vi "3Decembre2016.vi"() -> ()   [LabVIEW 2014]
panel:
  out "Nb de triangle Partie 2":dbl
  out "Nb de Triangles 4":dbl
  out "Nb de Triangles 3":dbl
  out "Nb de Triangles 2":dbl
  out "Nb de Triangles":dbl
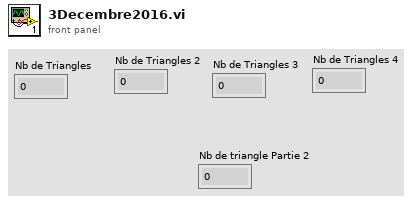
[diagram p1: front panel]
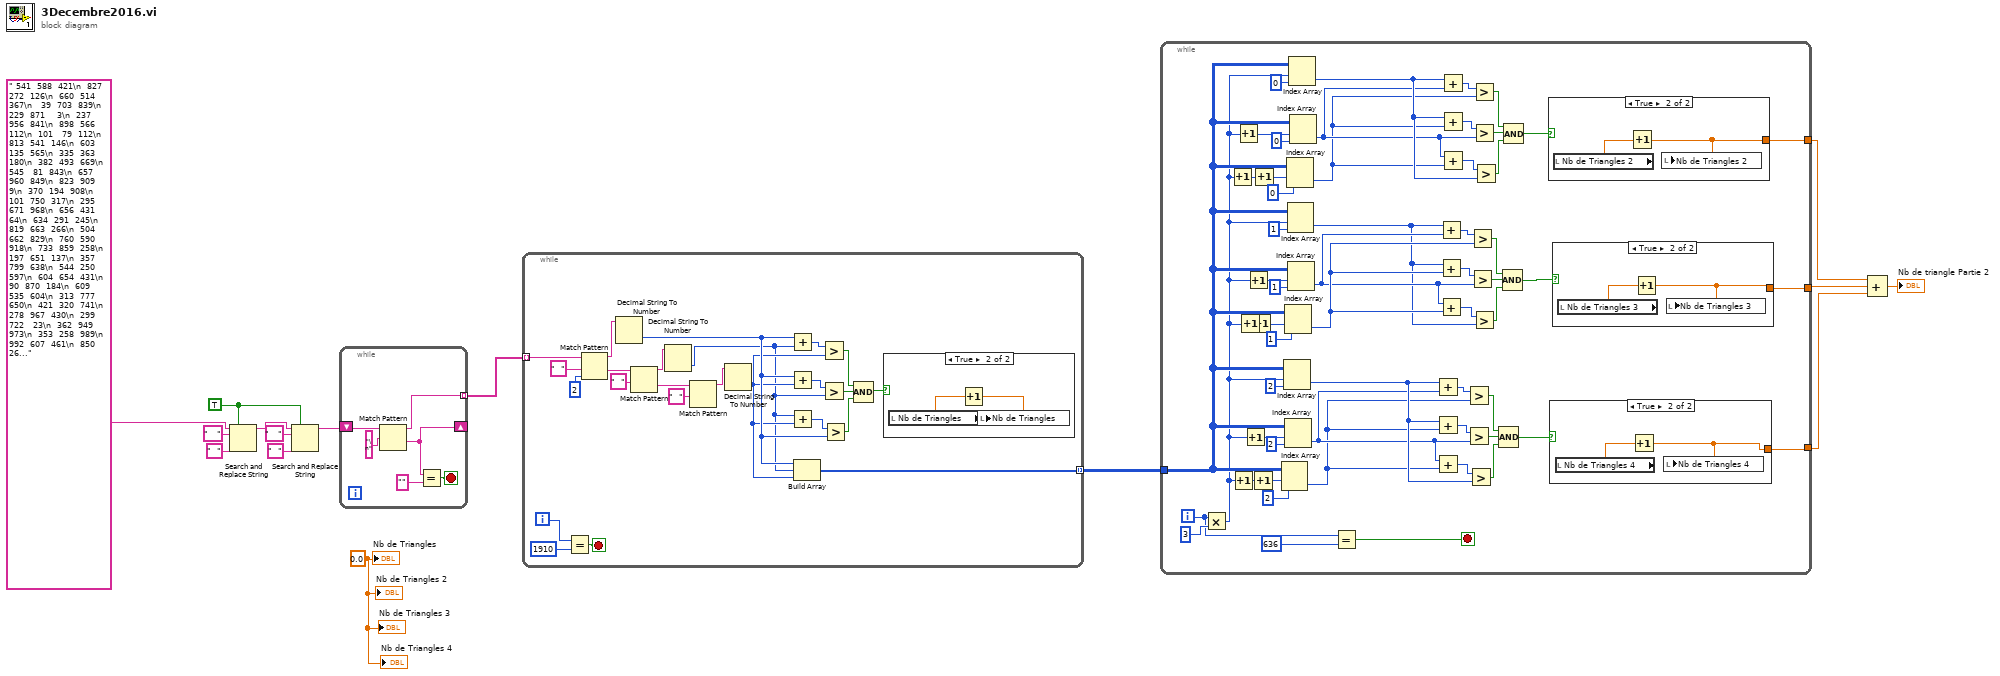
[diagram p0: block diagram]
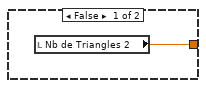
[diagram p2: hidden frame]
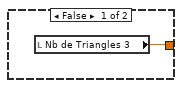
[diagram p3: hidden frame]
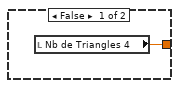
[diagram p4: hidden frame]
diagram:
  w1 = TRUE ("replace all? (F)")
  w14 = 0.0 ("Nb de Triangle")
  n1 = Search and Replace String(replace all?=w1, input string=" 541  588  421\n  827  272  126\n  660  514  367\n   39  703  839\n  229  871    3\n  237  956  841\n  898  566  112\n  101   79  112\n  813  541  146\n  603  135  565\n  335  363  180\n  382  493  669\n  545   81  843\n  657  960  849\n  823  909    9\n  370  194  908\n  101  750  317\n  295  671  968\n  656  431   64\n  634  291  245\n  819  663  266\n  504  662  829\n  760  590  918\n  733  859  258\n  197  651  137\n  357  799  638\n  544  250  597\n  604  654  431\n   90  870  184\n  609  535  604\n  313  777  650\n  421  320  741\n  278  967  430\n  299  722   23\n  362  949  973\n  353  258  989\n  992  607  461\n  850  264  490\n  251  351  569\n  810  320  116\n  959  335  611\n  450  242  624\n  849   26  376\n  419   42  222\n  995   14  291\n  711  174  615\n   17  982  961\n  722  895  941\n  920  161  480\n  905  246  531\n  794  190  144\n  317  318  633\n  145  233  150\n  445  534  519\n  935  592  863\n  784  260  844\n  255  704  570\n  521   57   61\n  490  149  110\n  163  144  142\n  771  289   60\n  914  233  541\n  271   93  542\n  411  640  812\n  370  968   65\n   61  960  781\n  333   79  421\n  269  190  428\n  477  225   96\n  610  641  265\n  650  135  461\n  145  759  380\n  758  451  682\n  524  125  861\n  760  555  251\n  360  219  567\n  456  285  726\n  510   98  927\n  886  336  228\n  356  916  323\n  685  974  165\n  253  532  207\n  868  990  548\n  811  803  525\n  205  624  894\n  707  512  328\n  835  288  657\n  496  776  413\n  484  185   10\n   33  832  403\n  896  678  789\n  745  595  773\n  287  201  669\n  150  189  513\n  884   42  131\n  934  214  407\n  239  819  149\n  145  582  334\n  375  307  467\n  680   59  850\n  873  441  973\n  243  393  256\n  509  237  265\n  302  550  334\n  728  524  291\n  130  986  333\n   60  926  390\n  133  653  692\n  428  755  491\n   24  476  659\n  446  290  823\n  906  703  410\n  950  183  391\n  199  735  250\n  734  908  254\n  635  373   34\n  489  567  275\n  587  746  463\n  512  508  367\n  104  971  568\n  647  857  191\n  605   20  775\n  118  853  634\n  432  559  322\n  887  433  134\n  660  332  336\n  669  711  952\n  762  713  610\n  108  972  860\n  732  743  562\n  877  277  758\n  225  590  380\n  708   35  424\n  989  425  439\n  279  413  818\n  107  422  634\n  775  833  667\n  755  755  279\n  694  293    6\n  156   75  649\n  820  303  651\n  448  934  587\n   25  830  788\n  473  192  932\n  734  126  535\n  940  215  513\n  935  126  656\n  428  905  789\n  760  742  772\n  510  523  633\n  994  808  110\n   93  740  100\n  943   80  198\n  329  888  532\n   50  763  337\n  320  673  741\n  722   52  639\n   18  130  566\n  733  130  921\n  280  586  642\n  450  222  350\n  178  427  325\n  317  685  261\n  744  261  105\n  621  809  326\n  740  532  605\n  855  690  526\n  441  301  185\n  783  309  196\n  525  272  334\n  502   58  432\n  980  150  121\n  891  9  800\n  286  143  705\n  985  846  850\n  362  696   70\n  807  194  900\n  912  193  448\n  405  148  461\n  677  261   30\n  121  406  308\n   34  206  451\n  109  473  312\n   46  726  695\n  793  847   25\n  834  160  708\n  372  849  375\n  744  799  423\n  631  478  715\n  346   82  545\n  541  184   95\n  492  228  588\n  542  635   43\n   75  347  439\n  612  321  431\n  719  526  847\n  158  270  338\n  813  482  560\n  817  253  402\n  899  630  887\n  198  456  730\n  235  286  344\n  125  646  398\n  204  375  401\n   80  289  308\n  295  664  862\n  284  382  565\n  816  130  651\n  947  596  383\n  131  611  723\n  617  471  549\n  663  282  697\n  475  219  901\n  535  829  434\n  542  502  544\n   23  649  110\n  733  691  820\n  684   21  821\n  740  689    1\n  224  249  280\n  485  776  350\n  682  971  182\n  465   12  610\n  294  296   13\n  606  297  594\n  337  104    3\n  154  257  343\n  352  171  349\n  322  466  973\n  189  173  854\n  484  338  714\n  194  194  551\n  188  741  162\n   14  696  663\n  219  868   33\n  224  4  446\n  218  865  411\n  392  536  574\n  616  692  482\n  746  592   94\n  230   72  663\n  291  487   99\n  326  482  669\n  131  265  155\n   61  422  609\n   80  552  641\n  509  334  851\n  475  211  911\n  193  274  737\n  128   15  973\n  381   31  255\n  413   21  812\n  778  461    3\n  514  307  697\n  329  353  695\n   48   90  212\n  856  354  294\n  863  265  360\n  496  918  264\n  377  889  164\n  603  164  418\n  159  701  199\n  283  503  186\n  127  658   54\n  938  226  855\n  189  533  465\n  924  365  906\n  322  422  291\n  943  713  238\n  714  508  138\n  612  328   49\n  962  877  685\n  849  963  732\n  154  278  428\n   49  624  476\n  111  518  753\n  284  330  216\n  716  689  290\n  667  369  127\n  719  728  175\n  543  493  139\n  759  408  286\n  915  970  827\n  482  289  787\n  713  860  621\n  836  286  729\n  921  447  223\n  665  655  706\n  692  579  316\n  772  679  289\n  972  394   84\n  221  675  877\n  272  336  864\n  439  684   69\n  780  721  503\n  225  587  125\n  802  945  408\n  280  237  682\n  406  281  745\n  176   60   71\n  450  720  335\n  656  293  383\n  324  694  454\n  547   57   51\n  415  965  657\n  311  936  687\n  989  878  585\n  156   72  165\n  938  823  574\n  626  968  146\n  823  896  588\n  294  236  597\n  177  294  177\n  287  351  480\n  133  252  649\n  706  319  175\n   34  418  960\n  722  583  906\n  711  379  674\n  529  574  882\n  546  868  781\n  577  875  687\n  881  844  503\n  926  247  190\n  621  535  356\n  294  105  257\n  601  640  579\n  573  142  519\n  978  900  427\n  693  823  350\n  275  362  683\n  137  291  741\n  258  130  517\n  838  686   12\n   59  800  869\n  790  188  881\n  997  324  278\n  582  338  887\n  900   23  712\n  288  619  402\n  480  168  596\n  292  505  505\n  993   30  982\n  636  335  892\n  813  363  175\n  230  248  620\n  450  668  896\n  460  736  874\n  331  800  837\n  844  805  734\n  620   54  708\n  726  820  592\n  126   20  394\n  728  820  219\n  229   27   32\n  164  569  939\n  290  559  949\n  325  360  794\n  342  356  529\n  203  627  691\n   60  932  544\n  767  865  563\n  770  316  525\n   99  756  674\n  165  783  180\n   72   27  846\n  973  419  905\n  104  364  294\n  896  271  613\n  294  222  416\n  414  609  858\n  481  429  478\n  308  544  615\n  624  139  560\n  574  626  840\n  998  338  328\n  403  739  211\n  625  472  120\n  808  190  64\n  5  202  558\n  800   42  607\n  874  801  675\n   27  275  735\n  898  927  280\n  366  794  526\n  233  529   13\n  314  744  525\n  842  530  617\n  704  461  406\n  281  946  841\n  389  113  678\n  545  652  410\n  851  754  339\n   14   56  706\n  623  131  738\n  636  127  931\n  857  404  199\n  682   25  387\n  574  406  435\n  508  528  307\n  574  531  575\n  223  433  827\n   80  811  486\n  710  642  904\n  749  903  795\n  920  205   60\n  904  286  108\n   96  428  120\n  631  364  307\n  599  169  180\n  743  491  302\n  133  939  980\n  559  879  883\n  642  605  918\n  935  868  810\n  539  860  357\n  584  643  972\n  831  562  800\n  211  561  108\n  953  928  802\n  730  611   73\n  483  373  139\n  245  374  210\n  493  582   77\n  671  422  887\n  568  458  930\n  727  462  467\n  663  603  657\n  113  490  966\n   95   26  415\n   74   84  463\n  117   78  276\n   81  814  741\n  407  852   36\n  348   39  748\n  144   43  826\n  915  174  218\n  775  148  820\n  388  305  131\n  458  135  195\n  142  199   96\n   79  223  625\n  338   47  879\n  295  217  575\n  790   72  723\n  713  736  711\n  366  769  330\n  302  642  718\n  603  526  956\n  450  181  663\n  176  638  433\n  902  801  408\n  750  545   97\n  398  366  271\n  490  186  474\n  801  290  324\n  964  652  190\n  937  593  344\n  112  888  373\n  940  377  623\n  668  693  367\n  623  889  870\n  231  714  220\n  694  535  837\n  701  178  674\n  620  887   23\n  603  133  576\n  224  983  601\n  3  103  234\n  867  232   33\n  869  235  233\n  448  909  262\n  247  941  265\n  464  909    4\n   30  224   22\n  154   99  764\n  146  187  786\n  789  347  512\n  474  166  775\n  583  253  359\n  517  531  274\n  154  414  735\n  397  436  997\n  864  822  104\n  712  303  243\n  310  652  217\n  915  772  521\n   25  780  616\n  927  266  233\n  899  327  372\n  796  897  343\n  741  794  508\n  533  554  586\n  470  656  176\n  159  863  749\n  680  644  839\n  784  768  143\n  152  451  939\n  125  366   67\n  779  902  437\n  657  749  452\n  325  759  722\n  576  562  249\n  776  467  790\n  776  580  296\n  705  264   84\n  522  526  220\n  879  278  392\n  712  426  442\n  288  589  363\n   74   23  960\n  203  873   22\n  170  857  952\n  155   46   56\n  840  855  211\n  740  816  188\n  644  272  737\n  623  362  311\n  309  416  848\n  895  807  900\n  196  790  127\n  871  912  916\n  569  966  180\n  461  223  854\n  805  754  886\n  828  353  453\n  263  697  656\n  595  541  418\n  235  302  908\n  883  446  723\n  996  745  204\n  457  813  925\n  674  271  977\n  463  769   97\n  668  535  957\n  609  720  417\n  889  987  722\n  649  852  317\n  450   69  383\n  499  915  226\n  430  185  435\n  475  840  992\n  775  992  695\n  334  725  933\n  642  273  908\n  682  693   55\n   14  532  444\n   63  192  736\n   51  362  930\n  306  301  474\n  448  330  373\n  691  115  425\n  431  321  623\n  265  881  504\n  591  726  138\n   58  930  870\n  540  954  120\n  496  157  772\n  116  376  817\n  943  249  828\n  945  384  518\n  777  573  897\n  769  254  676\n  290  691  734\n  845  818  135\n  860  802   75\n  956  267  157\n  964   92  268\n  631  126  262\n  571   59   14\n   45  226  368\n  144  878  306\n  166  940  581\n  803   30   24\n   40  408  268\n  782  423  267\n  511  251  426\n  680  962  467\n  919  817  103\n  558  609  789\n  619    7  544\n  122  611  384\n  503  449   80\n  373  982  264\n  355  559  207\n  911  801  105\n  382  889  894\n  762  707  989\n  754   83  383\n  890  198  327\n  189  185  492\n  844  820  374\n  602  375   81\n  399  871  374\n  576  446  620\n  696  249  930\n  203  510  741\n  485  264   79\n  485  310  443\n  163  340  469\n  187   15  873\n  309  506  141\n  319  508  753\n  202  457  500\n  560  614  177\n  377  909  534\n   84   32  898\n  261  761  825\n  207  763   85\n  649  544  761\n  874  639  578\n  760  555  435\n  738  108  970\n  711  458  986\n   31  529   83\n   98  374  182\n  344  620  186\n  421  340   29\n  490  860  153\n   97  793  609\n  412   70  510\n  855  542  805\n  753  320  429\n  130  245  621\n  173  309   23\n  741  513  716\n  588  632  728\n   53  928  543\n  429  868  480\n  455   90  465\n  673  302  632\n  238  255  483\n  455   49  181\n  325  935  570\n  631  118  140\n  579  987  515\n  385  485  576\n  466  497   16\n   85   57  595\n  967  801  619\n  792  543  386\n  842  480  332\n  861  688  780\n   88  209  741\n  784  542  396\n  696  800  232\n  434  969  747\n  709  342  679\n  698  892  147\n  526  474  726\n  491  707  679\n  241  197  440\n  799  371  452\n  832  425   98\n  249  288  669\n  657  909  768\n  657  930  957\n  751  211  846\n  2  642  844\n  748  718   11\n  694  764  366\n  332  231  268\n  580  593  459\n  921  656  751\n  171  757  815\n  828  555  167\n   38  409  765\n  244  455  834\n  251  121  421\n  659  271  526\n  401  470  326\n  354  241  846\n  145  732  473\n   53  261  972\n  192  594  511\n  480  337  383\n   68  182  937\n  472  478  653\n   84  346  471\n  707  458  137\n  710  483  366\n  954   52  537\n  871  116  778\n  670  104  912\n  989  639  346\n  139  444  640\n  876  497  599\n  313    8  980\n  211  896  163\n  127  894  850\n  504  230   28\n  385  710   79\n  602  553   90\n  981  628  560\n  653  532  914\n  452  275  432\n  251  486  366\n  521  257  539\n  385  255  892\n  552  405  361\n  220  223  576\n  608  368  309\n  287   92  647\n   33  346  483\n  271  397  213\n  834    8  851\n  450  129   51\n  477  139  847\n  652  619  430\n  525  117  446\n  505  656  250\n  387   34  263\n  288  651  381\n  450  665  145\n  704  612  710\n  875  974  543\n  887  419  378\n  328  768  521\n  249   30  936\n  318  762  906\n  807  242   71\n  794  413  374\n  100  200  330\n  317   65  889\n  268  175  870\n   69  215  691\n  487  484  583\n  368  497  505\n  402   64  263\n  290  420  846\n  552  525  839\n  300  497  485\n  371  144  551\n  590  391  504\n  790  519  261\n  533  533  519\n  997  537  453\n  869   26  534\n  179  787  612\n  470    6  559\n  407  781  138\n  239  498  490\n  390  291  976\n  604  227  556\n   78  937  610\n  513  171  447\n  528  874  853\n  308  925   92\n  113  114  109\n  286  820  150\n   68   64  664\n   29  952  167\n   86  988  736\n  530  285   93\n  533  829  394\n  654  917  322\n   79  802  748\n   79  226  476\n   63  681  810\n  699  249   37\n  970  116   99\n  332  355   71\n  821  366  189\n  653  531  751\n  577  791  917\n  841  104  877\n  717  993  919\n  342  969   58\n  469  458  501\n  190  446  208\n  511  151  600\n  635  875  369\n  443  580  620\n  235  761  902\n  170  707  130\n  404  586  241\n  270  920  319\n  280  340  126\n  226  357  857\n  432  401  816\n  122  962  518\n  903  139   38\n  886  928  553\n  884  636  522\n  139  696  787\n  936  455  611\n  935  238  617\n  879  265  631\n  162  490  358\n  447  520  570\n  283  118  375\n  432  411  768\n  468  110   89\n  642  116  624\n  299    8  687\n  426  802  789\n  428  846  419\n   21  750  486\n  306  251  164\n  824   54  144\n  625  273  242\n  625  507  776\n  618  429  200\n  7  81  763\n  167  288   97\n   60  239  173\n  223  370  259\n  719  160  934\n  895  833   51\n  961  693  984\n  240  940  566\n  240  869  930\n  171  457  848\n  105  693  480\n  807  288  493\n  839  883  538\n   18  659  905\n  883  665  543\n  904  746  659\n  225  119  529\n  523  104  507\n  447   57  109\n  642  234  709\n  319  554  656\n  849  437  597\n  648  645  614\n  482  447  953\n  891  321  883\n  432  423  391\n  295  684  242\n  214  303  540\n  562  256  130\n  784  369  960\n  414  510  954\n  395  508  442\n  790  536  212\n  764  463  384\n  515   37  205\n  857  840  421\n  778  876  558\n  594  698  882\n  274  425  847\n  463  766  592\n  825  456  751\n   42  530  818\n  800  812  238\n  795  832  365\n  879  814  318\n  102  763  445\n  916  349  731\n  165  838  485\n  757  973  270\n  520  501  512\n  682  157  411\n  326  563  238\n  881  173  303\n  776  160  358\n  810  284  156\n  169  981  827\n  132  886  635\n  109  223  359\n  785   28  287\n  2  855  288\n  782  854   23\n  824  452  743\n  425   79  768\n  839  380  810\n  859  212  356\n  545  250  389\n  341  270   90\n  271   31  500\n  958   38  718\n  890    7  642\n  437  869  750\n  267  488  241\n  481  517  781\n  898  751  423\n  363  244    7\n  938  960  415\n  714  297  426\n  821  370  697\n  454   77  498\n  290  171  296\n  257  509  698\n  504  455  525\n  619  771  981\n  502  179  779\n  554  746  322\n  554  203  273\n  576  557   27\n  560  474  284\n   76   85   88\n  366  418  956\n  426  487  928\n  468  783  402\n  547  167  678\n  206  627  728\n  467  191  185\n  621  856  989\n  618  794  862\n  183  667  714\n  582  707  993\n  558   38  366\n  324  111  131\n  939  660  600\n  863  576  550\n  761  410  470\n  414  273  362\n  411  148  179\n  532  795  514\n  299  214  719\n  296  871  522\n  557  895   97\n  489  873  782\n  398   81  760\n  493   75  328\n  832  502   96\n  482  505  247\n  378  667   38\n  463  434   78\n  190  789   78\n  798  510  131\n  855  502  824\n  698  775  920\n  685  930  693\n  920  723  923\n  911  303  901\n  668  574  538\n  8  832  573\n  670  629  626\n  248  686   96\n  434  131  743\n  456  716  679\n  294  807  107\n  533  284  167\n  765  615  130\n  958  870  257\n  910  169  662\n  304  829  425\n  600  235  796\n  411  788  121\n  243  840  791\n  576  707  927\n  613  307  633\n   58  888  639\n  634  707  253\n  589  371  730\n  193  956  813\n  733  551  197\n  155  973  175\n  763  477  200\n  102  984   83\n  207  427  487\n  135  868  546\n  375  596  389\n  329  405  299\n  496  691  230\n  266  975  261\n  295  834  423\n   80  140  572\n  844  660  625\n  772   44  369\n  171  642  782\n  352  889  273\n  788  228  588\n  737  852  753\n  599  322  664\n  545  296  545\n  445  137  454\n  218   69  171\n  234  928  681\n   67  991  829\n  166  131  174\n  442   11  769\n  324  133  795\n  736  757  408\n   49  177  439\n  719  923   31\n  497  953  502\n  664  684  447\n  173  497  278\n  954  888  913\n  764  118  107\n  601  850  972\n  466   61   19\n  969  499  418\n  686  460  404\n  327  329  165\n  596  726  139\n  811  596   75\n  185  331  327\n  216  409  168\n  160  196  483\n  264  533    1\n  227  495  151\n  226  708  155\n  580  345  615\n  586  900  862\n   16  699  871\n   38  594  382\n  760  684  141\n  770  455  511\n  286  821  117\n  582  919  393\n  433  979  346\n   75  939  949\n  102  899  631\n   98  305  567\n  349  636  399\n  627  981  520\n  948  639  181\n  753  150  521\n  776  563  328\n   89  613  658\n  552  747  504\n  131  449  276\n  429  824  391\n  283  542  472\n  731  199  435\n  456  707  160\n  675  243  107\n  547  911  854\n  170  849  912\n  497  869  377\n  475  951  392\n  458  273   24\n  140  109  311\n   38  276  388\n  151  274  515\n  100  704  858\n  811  362   42\n  745  777  817\n  740  497   81\n  424  270  266\n  375  714  277\n  602  668  923\n   33  492  225\n  603  953  772\n  244   65  920\n  247  659   29\n  380  651  916\n  674  529  388\n  656  624  288\n   53  112  270\n  653  385  841\n  736  945  725\n  474  883  204\n  995   21  127\n  264  886  337\n  873  870  237\n  275   42  834\n  188  202  872\n  232  234  490\n  688  384   29\n  713  174  281\n   90  533  299\n  365  437  364\n  345  940  484\n  572  829  274\n  556  319   28\n  310  736   27\n  758  729   19\n  919  993  823\n  942  949  411\n  520  610  663\n  376   24  997\n  876  668  790\n  762  682  677\n  530  224  905\n  480  624  428\n  127  796  916\n  777  114  158\n   38  824  844\n  771  821  741\n  870  738  438\n  615   13  677\n  856  751  710\n   68   89  515\n  827  390  728\n  889  356  930\n  741  935  128\n  858  515  386\n  641  922  307\n  714  383  434\n  381  638  194\n  710  290  388\n  601  658  846\n  610  559  781\n   10  439  810\n  114  699  864\n  848  860  733\n  949  736  155\n  454  185  588\n  188  877  350\n  597  820  593\n  240  725  614\n   22  553  516\n  239  428  318\n  707  173  296\n  649  766   51\n  557  760  313\n  913   62  485\n  362   24  684\n  805   55  212\n  610  397  255\n  331  680  376\n  733  339  525\n  777    7  686\n  879  920  684\n  495  926   25\n  175  533  818\n  678  810  343\n  690  823  682\n   52  185  180\n  245  228  826\n  299  102  977\n  904  227  871\n  867   20  889\n  666  220  171\n  696  805  515\n  380  681  837\n  738  243  339\n  576  513  714\n  898  609  914\n  732  403  842\n   65   29  417\n  635  604  578\n  588  610  339\n  123  147  654\n   65   80  660\n  113  123   70\n  530  767  183\n  154  253   34\n  377  994  217\n  991  771  825\n  557  595  223\n  839  175  698\n  680  414  626\n   57  876  930\n  675  735  408\n  674  747  543\n  547  749  929\n  161   36  383\n  286  951  733\n  453  923  535\n  480  575  661\n  643  402  847\n  630  953  624\n   21  888  632\n  136  814  335\n  833  441  246\n  937  388  147\n  613  604  255\n  668  625  410\n  196  660  255\n  117  333  779\n  884  780  853\n  912  919  303\n   72  632  889\n  929   27  933\n  858  630  181\n  647  439  851\n  543  205  795\n  270  431  312\n  514  300  234\n  455  290  594\n  415   38  755\n  392  749  796\n  760  749  105\n  368   10  783\n  844  620  117\n  514  323  208\n  359  499  126\n  641    9  263\n  636  233  362\n   61  245  109\n  665  493  989\n  494  711  865\n  195  534  431\n  200  651  721\n   42  832  577\n  178  262  431\n  912  555  708\n  891  524  503\n  326  978  344\n  984  371   44\n  678  443  935\n  655  654  905\n  384  602  298\n  828  716  458\n  734  243  645\n  200  588  627\n  434  319  449\n  541  648  208\n  618  393  505\n   49   51  527\n  651  431   27\n  794  116  242\n  454   99  190\n  614  169  369\n  635  347  837\n  533  718   55\n  127  859  890\n  809  535  303\n  922  487  246\n  199  619   78\n  124  599  113\n  951  248  547\n  853  792  528\n  639  270  510\n  704  256   49\n  192  143  521\n  821    5  339\n   14  299  920\n  827  296  810\n  396  630   54\n  409  319  535\n  582  850  483\n  748  125  175\n  876   51  329\n  536  141  309\n  944  357  396\n  807  390  188\n  889  577  474\n  778  295  217\n  752  299  217\n   45  424  155\n  506  283  758\n  239  427  742\n  740  162   16\n  103  466  204\n  656  718  395\n  711  370  556\n  915  240  466\n  381  152  564\n  698  136  118\n  801  989  979\n  404   20  740\n  920  980  503\n  426  449  642\n  345  396   63\n  314   52  601\n  908  910  453\n  639  943  749\n  886  903  652\n  505  623  394\n  564  131  304\n  250  542  119\n  470  353  683\n  207  558  664\n  587  282  129\n  368  850  270\n  721  525  763\n  857  515  929\n  163  172  921\n  813  379  716\n  848  308  879\n  231  683  824\n  564  715  305\n  589  903  967\n  452  576  371\n  120  820  215\n  444  536  215\n  897  300  478\n  659   78  489\n  688  259  807\n  475  744  132\n  430   47  721\n   59  729  594\n  123  255  846\n  267  822  141\n  283  982  920\n  914  670  772\n   31  803  762\n  882  940   22\n  196  889  610\n  412  540  310\n  473  467  599\n  186  108  628\n  749  266  559\n  876  263  736\n  741  794  155\n  916  489  217\n  244  683   93\n  735   32  860\n   79  469  774\n  694  498  168\n  875  971  968\n   44  660  936\n  891  909   68\n  335  803  447\n  592  440  192\n  602  625  528\n  964  299  913\n  864  165  676\n  870  211  388\n  139  658  896\n  161  710  828\n  239  681  111\n   71  727  871\n  899  324  898\n  876  969   47\n  102  426  768\n  645  531  788\n  740  143   24\n  126  687   39\n  692  236  701\n  680  904  696\n   19  888  694\n  315  353  457\n  331  917  500\n  407  291  968\n  335  410  880\n  558  515  406\n  450  379  766\n  500  149  685\n   90  442  254\n  590  573  807\n  444  759  934\n  547  983  229\n  591    6  764\n  457  631   82\n  351  623  791\n  697  240  380\n  680  586  523\n  142  542  564\n  196  568  103\n  671  672  588\n  861  102  540\n  297  946  373\n  351  757  750\n  573  445  421\n  110  931  491\n  244  667  417\n  253  852  662\n  133  258  885\n  801  791  404\n  840  867  890\n  138  506  521\n  786  496  173\n  813  618  607\n   56  189  183\n  143  464  143\n  194  568  251\n  553  975   89\n   40  956  336\n  529  579  340\n  517  876  870\n  698  748  771\n  513  191  220\n  985  754  351\n  297  869  155\n  865  124  214\n  349  627  737\n  458  241  398\n  383  417  996\n  469   56  636\n  281  379  667\n  290  375  403\n   61   54  128\n   47  999  378\n   16  996  484\n  453  718  314\n  324  643  418\n  240  134  361\n  890    9  340\n  141   90  353\n  868   94  582\n  876  486  539\n  231  662  114\n  981  831  580\n  609  264  435\n  510  378  388\n  125  321  143\n  245  785  782\n  171  368  238\n   78  959  740\n  174  264  202\n  797  597  391\n  832  496  415\n  155  676  108\n  648  947  171\n  630  556  239\n   75   61  727\n  356  439  740\n  363  455  230\n  746   64  703\n  699  487  178\n  110  477  537\n  347  640  201\n  704  118  559\n  857  719  453\n  215  861  623\n  665  768  311\n  635   95  630\n  418  547  323\n  546  432  466\n  635  256  163\n   20  948  990\n  164  982  281\n  152  173  745\n  688  580  193\n  602  239  331\n  875  390  312\n  935  818  360\n  163  996  778\n  838  617  720\n   69  195  442\n  795  604  370\n  809  647  473\n  724  606  742\n  709  743  861\n  101  798  285\n  656  333   91\n  541  591   94\n  185  327  149\n  677   34  945\n  543  170  473\n  544  183  994\n  578  574  351\n  560  863  386\n   62  613  114\n   67  950  242\n  303  606  171\n  364  461  152\n  592  209  521\n  736  696  587\n  935  534  284\n  466  283  120\n  301  458  742\n  622  618  758\n  332  643  475\n  704  495  412\n  386  920  113\n  632  658  906\n  405  917  669\n  969  309  974\n  762   93  102\n  778  191  601\n  897  117  681\n  313  553  678\n   60  703  504\n  360  711  335\n  240  415  317\n   83  256  292\n  182  622  509\n  945  298  318\n  812  581  650\n  988  778  820\n  744  692  625\n  808  652   11\n  156  285  613\n  256   59  486\n  9  493  462\n  246  488  875\n  476  284  372\n   84  413  124\n  508  626  464\n  784  760  569\n  275  439  701\n  669  705  634\n  571  647  526\n  704  798  866\n  141  939  981\n  700  416  888\n  677  579  687\n  127  250  564\n  302  288  392\n  747  164  661\n  876  145  974\n  235  776  950\n  698  425   25\n  711  960  937\n  587  155  168\n  321   39  529\n  843  172  601\n  538  979   79\n  209  788  585\n  347  615  623\n  605  703   53\n  348  760  293\n  825  194  336\n  246  913  550\n  571  745  359\n  755  305  568\n  137  502  612\n   92  335  819\n  185  176  244\n  793  927  516\n   90  917   10\n  795  120  526\n  376  200  481\n  935  286  222\n  745  116  477\n  132  528  588\n  812  162  598\n  926  516   67\n  137  753  113\n  762  860  967\n  894  663  993\n  420  933  587\n  822  614  897\n  946  964  988\n  731  224  756\n  582  547  763\n  273  333   12\n  520  794  181\n  461  498  846\n  970  493  885\n  866  400  229\n  895  427  943\n   80  303  913\n  658  256  244\n  481  981  281\n  418  784  512\n  785  739  556\n  598   79  548\n  905  798   18\n   16  747  709\n  604  422  109\n  622  337  607\n  235  664  940\n  192  928  263\n  427  669  747\n  259  364  794\n  312  606  973\n   66  888  604\n  504  601  128\n  789  731  543\n  883  385  584\n  549  746  739\n  243   30  974\n  517  774  893\n  479  361  847\n  507  170  333\n  264  387  860\n  688  905  485\n  302  677  369\n  521  918  694\n  306  435  744\n  413  683  692\n  662  504  471\n  131  393  765\n  277  613  541\n  311  977  448\n   77  714  200\n  535  760  407\n  567  910  371\n  477  161  408\n  175  224  834\n  524  139  423\n   53  197  234\n  741   44  130\n  747  220  343\n  152  970  844\n  517  178   54\n  585  864  867\n  812  201   16\n  434  561   27\n  617  372   23\n  483  981  131\n  635  157  182\n  729  836  185\n  638  762  607\n   99  836   79\n  714  939  613\n   19  369  171\n  168  424  312\n  161  605  447\n  294   24  766\n  390   16  992\n  188   31  532\n  876  971  282\n  893  980  505\n   36   64  438\n  820  658  792\n  784  742  672\n  544  951  415\n  825  586  313\n  115   47  298\n  913  539  539\n  399  383  574\n  5  616  775\n  401  574  837\n  932  186  210\n  314  140  652\n  685   75  667\n  683  303  224\n  654  260  698\n  269  338  909\n  481  395  983\n  467  651  337\n  117  633  789\n  960  676  402\n  570  438  248\n  537  686  151\n  100  375  563\n  894  196  476\n  902  430  890\n  832  161  413\n  852  600  150\n  655  713  277\n  223  462  773\n  579  348  861\n  423  599  107\n  820  655  872\n  664  615  487\n  175  158  793\n  382  330  208\n  226  433  657\n  316  321  505\n  332  718  917\n  349  349  837\n  220  449  309\n  353   49  699\n  745  314  852\n  488  295  161\n  390  277  913\n  403  130  139\n  194  244  874\n  250  900  126\n  234  800   17\n  434  407  144\n  502  334  514\n  777  558  417\n  581  435  444\n  644  399  448\n  351  674  351\n  588  789  785\n  418  283  642\n  410  177  125\n  110  116  747\n  116  392  639\n   22  250  219\n  106  332  452\n  882  523  655\n  838  798  712\n  970  438   99\n  796  526  268\n   18  569  586\n  811  154  770\n  225  483  638\n  700  365  856\n  628  121  280\n  109  217   93\n  610  365  262\n  628  309  184\n  716  382  175\n   72  480  116\n  762  852   94\n  398  119  308\n  595  323  380\n  289  260  116\n   73   26  147\n  833  574  967\n  790  595  890\n  513  446  883\n  657  520  594\n  241  206  421\n  193  383  465\n  993  932  141\n  972  902  489\n   54  459  409\n   67  134  614\n   43  487  631\n  578  500  479\n  728  426  182\n  441  202  325\n  213  653  761\n  311  499  642\n  265  939  467\n  457  609  840\n   43  732  121\n  487  317  958\n  223  424  394\n  489  429   40\n  367   87  362\n  420  217   87\n  628  855  185\n  212  679  162\n  142  146  150\n  770  529  597\n  735  410  568\n  457  497  182\n  203  447   45\n  266  299  200\n  933  580   14\n  345  883  795\n  629  311  798\n   81  312  674\n   25   40  629\n   58  343   43\n  285  384  381\n  365  202  764\n  144  319  775\n  236  237  727\n  219  681  491\n  374  901  870\n  429   92   77\n  561   73  648\n  845   28  647\n  764  497  183\n  345  591   73\n  824  804  193\n   37  452  516\n   12   25  584\n   33  431  562\n  283  354  846\n  457  278   67\n  698  201  894\n   26  283  646\n  658  597  344\n  686  455  490\n  473  265  560\n  497  207  736\n  140  298  623\n  588  960  698\n  591   32  249\n  3  973  823\n  265  151  789\n  644  300   86\n  552  366  744\n  561  302  955\n  547  867  988\n  514  852  638\n  682  499  416\n  573  945  845\n  535  635  658\n  197  495  330\n  333  483  690\n  309   42  532\n  489  158  372\n  566  482  961\n  109  341  783\n  677  712  119\n  531   37  232\n  340  720  347\n  913  134  690\n  889  142  429\n  206  232  821\n  742  721  309\n  461  532  188\n  888  360  389\n  671  950  531\n  569  238  573\n  205  837  461\n  678  911  560\n  537  935  552\n  245  346  500\n   84  225  546\n  506  752  793\n  499  609  383\n  246  199  476\n  197  634  991\n  420  554  641\n  238  720  826\n  571  179  321\n  547  902  890\n  550    5  156\n  424  149  875\n  598  156  814\n  724   95  766\n   38  236  620\n  742  238  162\n  462  213  218\n  283  599  565\n  460  812  473\n  331  733  798\n   43   32  896\n  286  711  908\n  406  288  678\n  515  881  387\n  914  756  617\n  300  178    3\n  559  543  905\n  485  486  909\n  851  950  411\n  360  806  419\n  704  305  747\n  730  206   61\n  808  435  421\n  588  349  416\n  346  519  684\n  718  771  253\n  936  695  748\n  966  123  346\n  487  571  976\n  717  673  998\n  343  505  124\n  109  169  918\n  247  646  985\n  850  995  239\n  702  762  661\n  733  677  459\n   54  660   25\n  625  661  192\n  654   55  168\n  227  364  350\n  221  655  867\n   52  413  767\n  948  714  641\n  111  412  816\n  859  833  382\n  250  719  818\n  528  616   94\n  386  203  781\n  111  447  244\n  316  383  677\n  280  100  824\n  452  322  649\n  634  793  332\n  625  665  349\n   49  435  758\n  320  580  776\n  352  166  227\n  691  801  376\n   89  794   10\n  758   19  387\n   24  951  738\n  584  127  681\n  564  888  469\n  421  813  308\n  120  380  894\n  539  675  908\n  610  112  430\n  605  196  435\n  822   89   10\n  912  760  205\n  497  850  873\n  472  876  699\n  582  896  978\n  727  238  974\n  748  784  223\n  961  411  965\n  954  767   62\n  148  855  987\n  832  955  512\n  399  748  110\n  530  616  422\n  525  708  992\n  668  340  962\n  833  804  120\n  797  294  259\n  693  181  688\n  898  165  715\n  675  424  309\n  596   76  129\n  519  470  267\n  377  926  744\n  551   66  834\n  560  976  275\n  475  551   92\n  195  468  205\n  446  358  122\n  366  338  734\n  972  710  760\n  914  818   24\n  532  324  333\n   75  917  277\n  605  656  369\n  727  548  469\n   58   84  437\n  674  524   68\n  467  452  792\n  841  519  660\n  922  861  946\n  682  753  605\n  777  419  758\n  536  434  269\n  291  624  351\n  372  151  768\n   86  579  751\n  252  720  474\n  976  739  949\n  878   23  771\n  320  259  561\n  536  887  709\n  491  828  668\n  949  488  913\n  973   40  122\n  868  492  808\n  261  938  614\n   42  327  679\n  296  806  227\n  251  681  523\n  555  933  543\n  802  343   31\n  739  605  863\n  581  553  337\n  198  880  885\n  139  466  781\n  479  471  785\n  565   29   36\n  962  283  367\n  756  881  927\n  761  837  936\n  413  712  289\n  118  620   91\n  297  732  256\n  733  895  489\n  163   12  540\n  655  898  321\n  241  509  371\n  916  272  653\n  688  281  810\n  103  215  281\n  987   92  408\n  957  170  454\n  466   88  293\n  40  813  103\n  436  766  254", search string="   ", replace string="  " ("replace string (\"\")")) -> (result string=w4:string)  [unwired: 4 in, 3 out]
  n2 = Search and Replace String(replace all?=w1, input string=w4, search string="   ", replace string="  " ("replace string (\"\")")) -> (result string=w5:string)  [unwired: 4 in, 3 out]
  n3 = while {
    shift-right: [w17] -> _
    shift-left: w5 -> [w21]
    tunnel: [w19] -> w15 mode=indexing
    stop <- w18 stop-if-true
    n4 = Match Pattern(string=w21, regular expression="\n") -> (before substring=w19:string, after substring=w17:string)  [unwired: 1 in, 2 out]
    n5 = Equal?(x=w17, y="") -> (x = y?=w18:bool)
  }
  n6 = while {
    tunnel: w15 -> [w41] mode=indexing
    tunnel: [w23] -> w2 mode=indexing
    i -> [w35]
    stop <- w45 stop-if-true
    n7 = Equal?(x=w35, y=1910) -> (x = y?=w45:bool)
    n8 = Match Pattern(string=w41, regular expression="  ", offset (0)=2) -> (before substring=w39:string, after substring=w40:string)  [unwired: 2 out]
    n9 = Decimal String To Number(string=w39) -> (number=w25:i32)  [unwired: 2 in, 1 out]
    n10 = Match Pattern(string=w40, regular expression="  ") -> (before substring=w37:string, after substring=w36:string)  [unwired: 1 in, 2 out]
    n11 = Decimal String To Number(string=w37) -> (number=w22:i32)  [unwired: 2 in, 1 out]
    n12 = Match Pattern(string=w36, regular expression="  ") -> (before substring=w26:string)  [unwired: 1 in, 3 out]
    n13 = Decimal String To Number(string=w26) -> (number=w24:i32)  [unwired: 2 in, 1 out]
    n14 = Add(x=w25, y=w22) -> (x+y=w33:i32)
    n15 = Add(x=w25, y=w24) -> (x+y=w32:i32)
    n16 = Add(x=w22, y=w24) -> (x+y=w31:i32)
    n17 = Build Array(w25, w22, w24) -> (w23:i32[])
    n18 = Greater?(x=w33, y=w24) -> (0:w29:bool)
    n19 = Greater?(x=w32, y=w22) -> (0:w30:bool)
    n20 = Greater?(x=w31, y=w25) -> (0:w28:bool)
    n21 = Compound Arithmetic op=AND(w29, w30, w28) -> (w27:bool)
    n22 = case shown="True" w27 {
      frame False {
      }
      frame True {
        n23 = local read "Nb de Triangles"() -> (w46:dbl)
        n24 = Increment(x=w46) -> (x+1=w47:dbl)
        n25 = local write "Nb de Triangles"(w47) -> ()
      }
    }
  }
  n26 = while {
    tunnel: w2 -> [w74]
    tunnel: [w52] -> w12
    tunnel: [w51] -> w11
    tunnel: [w50] -> w13
    i -> [w54]
    stop <- w48 stop-if-true
    n27 = Multiply(x=w54, y=3) -> (x*y=w55:i32)
    n28 = Increment(x=w55) -> (x+1=w66:i32)
    n29 = Increment(x=w55) -> (x+1=w69:i32)
    n30 = Increment(x=w55) -> (x+1=w67:i32)
    n31 = Increment(x=w55) -> (x+1=w72:i32)
    n32 = Increment(x=w55) -> (x+1=w70:i32)
    n33 = Increment(x=w55) -> (x+1=w73:i32)
    n34 = Increment(x=w72) -> (x+1=w71:i32)
    n35 = Increment(x=w69) -> (x+1=w68:i32)
    n36 = Increment(x=w66) -> (x+1=w65:i32)
    n37 = Index Array(array=w74, index (row)=w68, index (col)=2 ("disabled index (col)")) -> (element=w49:i32)
    n38 = Index Array(array=w74, index (row)=w55, index (col)=2 ("disabled index (col)")) -> (element=w96:i32)
    n39 = Index Array(array=w74, index (row)=w71, index (col)=1 ("disabled index (col)")) -> (element=w94:i32)
    n40 = Index Array(array=w74, index (row)=w70, index (col)=2 ("disabled index (col)")) -> (element=w95:i32)
    n41 = Index Array(array=w74, index (row)=w65, index (col)=0 ("disabled index (col)")) -> (element=w75:i32)
    n42 = Index Array(array=w74, index (row)=w55, index (col)=1 ("disabled index (col)")) -> (element=w92:i32)
    n43 = Index Array(array=w74, index (row)=w73, index (col)=1 ("disabled index (col)")) -> (element=w93:i32)
    n44 = Index Array(array=w74, index (row)=w55, index (col)=0 ("disabled index (col)")) -> (element=w77:i32)
    n45 = Index Array(array=w74, index (row)=w67, index (col)=0 ("disabled index (col)")) -> (element=w76:i32)
    n46 = Equal?(x=w54, y=636) -> (x = y?=w48:bool)
    n47 = Add(x=w96, y=w95) -> (x+y=w103:i32)
    n48 = Add(x=w96, y=w49) -> (x+y=w102:i32)
    n49 = Add(x=w95, y=w49) -> (x+y=w101:i32)
    n50 = Add(x=w92, y=w93) -> (x+y=w86:i32)
    n51 = Add(x=w92, y=w94) -> (x+y=w87:i32)
    n52 = Add(x=w93, y=w94) -> (x+y=w88:i32)
    n53 = Add(x=w77, y=w76) -> (x+y=w83:i32)
    n54 = Add(x=w77, y=w75) -> (x+y=w82:i32)
    n55 = Add(x=w76, y=w75) -> (x+y=w81:i32)
    n56 = Greater?(x=w103, y=w49) -> (0:w99:bool)
    n57 = Greater?(x=w102, y=w95) -> (0:w100:bool)
    n58 = Greater?(x=w101, y=w96) -> (0:w98:bool)
    n59 = Greater?(x=w86, y=w94) -> (0:w90:bool)
    n60 = Greater?(x=w87, y=w93) -> (0:w89:bool)
    n61 = Greater?(x=w83, y=w75) -> (0:w79:bool)
    n62 = Greater?(x=w82, y=w76) -> (0:w80:bool)
    n63 = Greater?(x=w88, y=w92) -> (0:w91:bool)
    n64 = Greater?(x=w81, y=w77) -> (0:w78:bool)
    n65 = Compound Arithmetic op=AND(w99, w100, w98) -> (w104:bool)
    n66 = Compound Arithmetic op=AND(w90, w89, w91) -> (w85:bool)
    n67 = Compound Arithmetic op=AND(w79, w80, w78) -> (w84:bool)
    n68 = case shown="True" w84 {
      tunnel: [w105 w106] -> w51
      frame False {
        n69 = local read "Nb de Triangles 2"() -> (w105:dbl)
      }
      frame True {
        n70 = local read "Nb de Triangles 2"() -> (w107:dbl)
        n71 = Increment(x=w107) -> (x+1=w106:dbl)
        n72 = local write "Nb de Triangles 2"(w106) -> ()
      }
    }
    n73 = case shown="True" w104 {
      tunnel: [w111 w112] -> w50
      frame False {
        n74 = local read "Nb de Triangles 4"() -> (w111:dbl)
      }
      frame True {
        n75 = local read "Nb de Triangles 4"() -> (w113:dbl)
        n76 = Increment(x=w113) -> (x+1=w112:dbl)
        n77 = local write "Nb de Triangles 4"(w112) -> ()
      }
    }
    n78 = case shown="True" w85 {
      tunnel: [w108 w109] -> w52
      frame False {
        n79 = local read "Nb de Triangles 3"() -> (w108:dbl)
      }
      frame True {
        n80 = local read "Nb de Triangles 3"() -> (w110:dbl)
        n81 = Increment(x=w110) -> (x+1=w109:dbl)
        n82 = local write "Nb de Triangles 3"(w109) -> ()
      }
    }
  }
  n83 = Compound Arithmetic op=ADD(w11, w12, w13) -> (→"Nb de triangle Partie 2":dbl)
  "Nb de Triangles" <- w14
  "Nb de Triangles 2" <- w14
  "Nb de Triangles 3" <- w14
  "Nb de Triangles 4" <- w14
